vi "SwerveJoystickLogic.vi"() -> (2 "Speeds":dbl[](array[numeric]), 3 "Angles":dbl[](array[numeric]))   [LabVIEW 2018]
uses:
  SwerveGlobals.vi
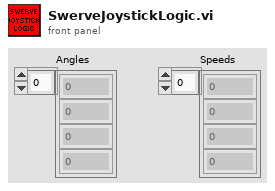
[diagram p1: front panel]
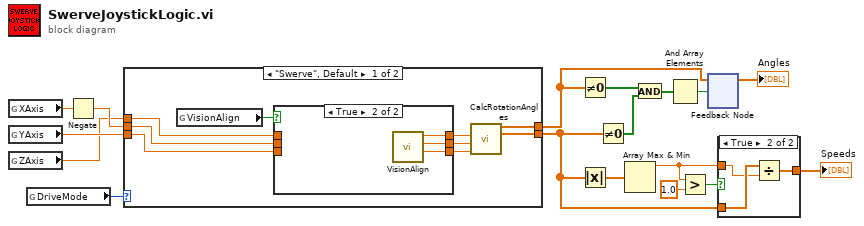
[diagram p0: block diagram]
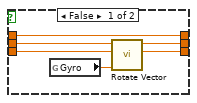
[diagram p3: hidden frame]
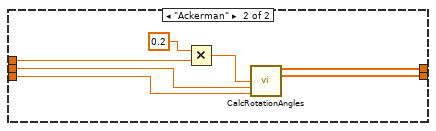
[diagram p4: hidden frame]
diagram:
  n1 = global read "SwerveGlobals.vi" "XAxis"() -> (w13:dbl)
  n2 = global read "SwerveGlobals.vi" "YAxis"() -> (w3:dbl)
  n3 = global read "SwerveGlobals.vi" "ZAxis"() -> (w2:dbl)
  n4 = global read "SwerveGlobals.vi" "DriveMode"() -> (w12:enum16{"Swerve", "Ackerman"})
  n5 = Negate(x=w13) -> (-x=w4:dbl)
  n6 = case shown="\"Swerve\", Default" w12 {
    tunnel: [w26 w38] -> w10
    tunnel: w4 -> [w23 w41]
    tunnel: w3 -> [w22 w40]
    tunnel: w2 -> [w24 w42]
    tunnel: [w25 w39] -> w6
    frame "Swerve", Default {
      n7 = global read "SwerveGlobals.vi" "VisionAlign"() -> (w20:bool)
      n8 = case shown="True" w20 {
        tunnel: [w32 w35] -> w21
        tunnel: w24 -> [w32 _]
        tunnel: [w28 w34] -> w19
        tunnel: w23 -> [w30 _]
        tunnel: [w27 w33] -> w18
        tunnel: w22 -> [w29 _]
        frame False {
          n9 = global read "SwerveGlobals.vi" "Gyro"() -> (w31:dbl)
          n10 = call "Rotate Vector.vi"("Angle"=w31, "Y"=w29, "X"=w30) -> ("Y'"=w27:dbl, "X'"=w28:dbl)  [unwired: 6 in]
        }
        frame True {
          n11 = call "VisionAlign.vi"() -> ("Y"=w33:dbl, "X"=w34:dbl, "Z"=w35:dbl)  [unwired: 9 in]
        }
      }
      n12 = call "CalcRotationAngles.vi"("ZAxis"=w21, "XAxis"=w19, "YAxis"=w18) -> ("Angles"=w25:dbl[], "Speeds"=w26:dbl[])  [unwired: 11 in]
    }
    frame "Ackerman" {
      n13 = Multiply(x=0.2, y=w42) -> (x*y=w37:dbl)
      n14 = call "CalcRotationAngles.vi"("ZAxis"=w37, "XAxis"=w41, "YAxis"=w40) -> ("Angles"=w39:dbl[], "Speeds"=w38:dbl[])  [unwired: 11 in]
    }
  }
  n15 = Not Equal To 0?(x=w6) -> (x != 0?=w8:bool[])
  n16 = Absolute Value(x=w10) -> (abs(x)=w14:dbl[])
  n17 = Not Equal To 0?(x=w10) -> (x != 0?=w7:bool[])
  n18 = Array Max & Min(array=w14) -> (max value=w15:dbl)  [unwired: 3 out]
  n19 = And(x=w8, y=w7) -> (x .and. y?=w11:bool[])
  n20 = And Array Elements(Boolean array=w11) -> (logical AND=w5:bool)
  n21 = Greater?(x=w15, y=1.0) -> (0:w17:bool)
  n22 = feedback #1() -> (→"Angles":dbl[])  [unwired: 1 in]
  n23 = feedback-in #1(w6, w5) -> ()
  n24 = case shown="True" w17 {
    tunnel: w10 -> [w43 w46]
    tunnel: w15 -> [_ w45]
    tunnel: [w43 w44] -> w1
    frame False {
    }
    frame True {
      n25 = Divide(x=w46, y=w45) -> (x/y=w44:dbl[])
    }
  }
  "Speeds" <- w1
